vi "False.vi"(0 "VI Reference In":refnum<vi>, 1 "Label":string, 2 "delimiter (>>)":string=">>", 3 "Assert Only? (F)":bool, 5 "Control Name":string, 11 "Error In":errorcluster, 12 "Assert Interval(10 ms)":u32=10, 13 "Timeout(5 sec)":dbl=5.0) -> (4 "VI Reference Out":refnum<vi>, 15 "Error Out":errorcluster)   [LabVIEW 2016, in "Drona.lvlib" / "AssertControlValue.lvlib"]
doc: "Asserts if the values of control is false.\n\nThe input control name is given as a string , incase of path, use delimiters inbetween the path.\nThis VI gets the value of the control, untill the value is false."
uses:
  AssertControlValue.lvlib
  Setup/GetControlRef/GetControlRefByPath.vi
  <vilib>/addons/_JKI Toolkits/Caraya/classes/Assert/Assert.lvclass
  Setup/GetControlRef/GetControlRef.lvlib
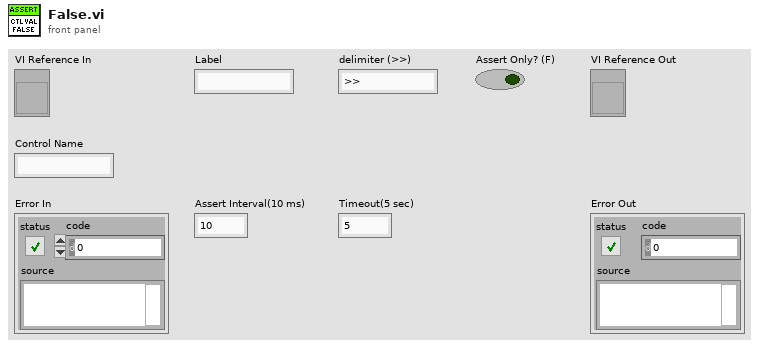
[diagram p1: front panel]
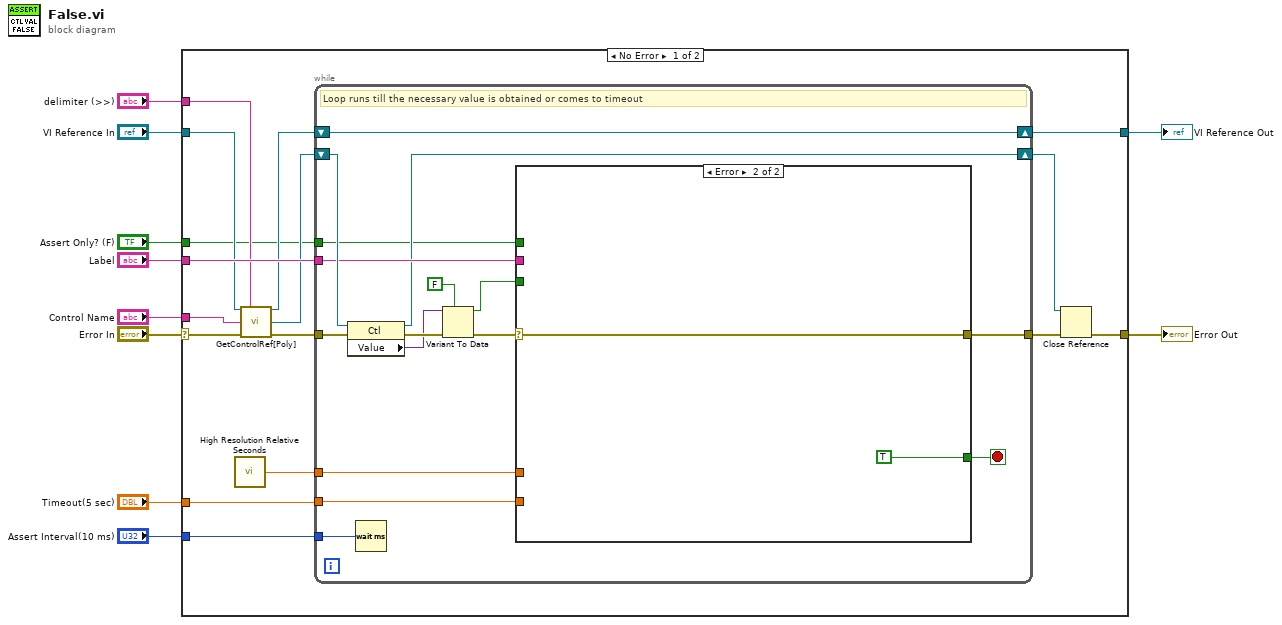
[diagram p0: block diagram]
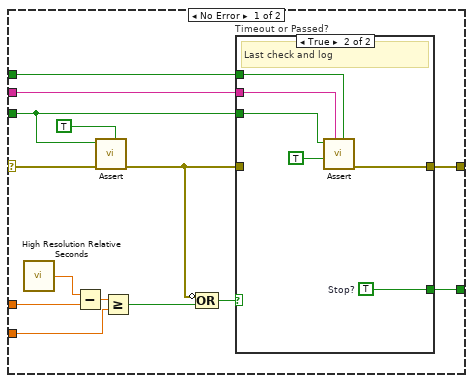
[diagram p2: hidden frame]
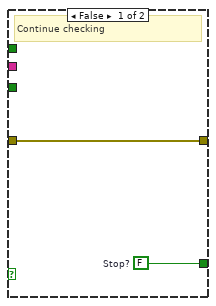
[diagram p3: hidden frame]
diagram:
  n1 = case shown="No Error" "Error In" {
    selector: "Error In" -> [w21 w68]
    tunnel: "Timeout(5 sec)" -> [w26 _]
    tunnel: [w25 w67] -> w9
    tunnel: [w14 w68] -> w8
    tunnel: "Assert Interval(10 ms)" -> [w23 _]
    tunnel: "Label" -> [w22 _]
    tunnel: "VI Reference In" -> [w20 w67]
    tunnel: "Control Name" -> [w19 _]
    tunnel: "delimiter (>>)" -> [w12 _]
    tunnel: "Assert Only? (F)" -> [w11 _]
    frame No Error {
      n2 = call <vilib>:"High Resolution Relative Seconds.vi"() -> ("relative seconds"=w18:dbl)
      n3 = call-poly "GetControlRef[Poly].vi"("VI Reference In"=w20, "delimiter (>>)"=w12, "Control Name"=w19, "error In"=w21) -> ("VI Reference Out"=w16:refnum<vi>, "Ctl Refnum"=w15:refnum<vi>, "error out"=w17:errorcluster)  [unwired: 9 in]
      n4 = while {
        tunnel: w26 -> [w41]
        tunnel: w18 -> [w42]
        tunnel: w17 -> [w36]
        tunnel: [w39] -> w24
        tunnel: w23 -> [w37]
        tunnel: w22 -> [w33]
        shift-right: [w34] -> w25
        shift-left: w16 -> [w34]
        shift-right: [w32] -> w13
        shift-left: w15 -> [w35]
        tunnel: w11 -> [w27]
        stop <- w40 stop-if-true
        # "Loop runs till the necessary value is obtained or comes to timeout"
        n5 = property class="Ctl"(reference=w35, error in=w36) -> (reference out=w32:refnum<vi>, error out=w38:errorcluster, "Value"=w30:variant)
        n6 = Wait (ms)(milliseconds to wait=w37) -> ()  [unwired: 1 out]
        n7 = Variant To Data(error in=w38, type=FALSE, Variant=w30) -> (data=w29:bool, error out=w31:errorcluster)
        n8 = case shown="Error" w31 {
          selector: w31 -> [w52 w66]
          tunnel: w42 -> [w56 _]
          tunnel: w41 -> [w53 _]
          tunnel: [w45 TRUE] -> w40
          tunnel: [w46 w66] -> w39
          tunnel: w29 -> [w44 _]
          tunnel: w33 -> [w51 _]
          tunnel: w27 -> [w43 _]
          frame No Error {
            n9 = call <vilib>:"High Resolution Relative Seconds.vi"() -> ("relative seconds"=w55:dbl)
            n10 = Subtract(x=w55, y=w56) -> (x-y=w54:dbl)
            n11 = call-poly <vilib>:"Assert.vi"("Assert Only? (F)"=TRUE, "error in (no error)"=w52, "False?"=w44) -> ("error out"=w49:errorcluster)  [unwired: 8 in]
            n12 = Greater Or Equal?(x=w54, y=w53) -> (x >= y?=w50:bool)
            n13 = Compound Arithmetic op=OR(invert w49, w50) -> (w48:bool)
            n14 = case "Timeout or Passed?" shown="True" w48 {
              tunnel: w49 -> [w58 _]
              tunnel: w44 -> [_ w63]
              tunnel: w51 -> [_ w64]
              tunnel: [w58 w62] -> w46
              tunnel: [w57 w61] -> w45
              tunnel: w43 -> [_ w59]
              frame False {
                w57 = FALSE  # Stop?
                # "Continue checking"
              }
              frame True {
                w61 = TRUE  # Stop?
                # "Last check and log"
                n15 = call-poly <vilib>:"Assert.vi"("Assert Only? (F)"=w59, "Label"=w64, "Register with caller test (F)"=TRUE, "False?"=w63) -> ("error out"=w62:errorcluster)  [unwired: 7 in]
              }
            }
          }
          frame Error {
          }
        }
      }
      n16 = Close Reference(reference=w13, error in (no error)=w24) -> (error out=w14:errorcluster)
    }
    frame Error {
    }
  }
  "Error Out" <- w8
  "VI Reference Out" <- w9
